vi "TPNT_GetDDSStream.vi"(10 "name in":string) -> (2 "name out":string)   [LabVIEW 2016]
uses:
  DBSHAND/private/vis/DatabaseHand_Element_Get(string).vi
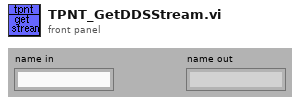
[diagram p1: front panel]
types:
  T1 = typedef "DatabaseHand_RefNum.ctl" = refnum<vi>
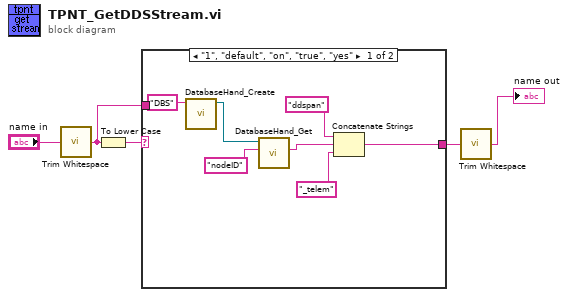
[diagram p0: block diagram]
diagram:
  n1 = call <vilib>:"Trim Whitespace.vi"("string"="name in") -> ("trimmed string"=w2:string)  [unwired: 1 in]
  n2 = To Lower Case(string=w2) -> (all lower case string=w3:string)
  n3 = case shown="\"1\", \"default\", \"on\", \"true\", \"yes\"" w3 {
    tunnel: [w6 w13] -> w5
    tunnel: w2 -> [_ w13]
    frame "1", "default", "on", "true", "yes" {
      n4 = call "DatabaseHand_Create.vi"("Name"="DBS") -> ("Database RefNum out"=w11:T1)  [unwired: 1 in, 9 out]
      n5 = call-poly "DatabaseHand_Get.vi"("name"="nodeID", "Database RefNum in"=w11) -> ("value"=w8:string)  [unwired: 3 in, 6 out]
      n6 = Concatenate Strings("ddspan" ("string"), w8, "_telem" ("string")) -> (w6:string)
    }
    frame Default {
    }
  }
  n7 = call <vilib>:"Trim Whitespace.vi"("string"=w5) -> ("trimmed string"=→"name out":string)  [unwired: 1 in]
